vi "GetHWinfobyWMIC.vi"() -> (1 "CPUID":string, 2 "BoardSN":string)   [LabVIEW 2015]
uses:
  <vilib>/regexp/Match Regular Expression.xnode
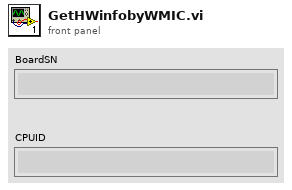
[diagram p1: front panel]
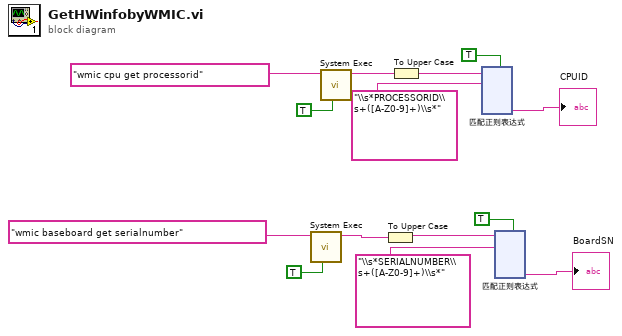
[diagram p0: block diagram]
diagram:
  n1 = call <vilib>:"System Exec.vi"("run minimized? (F)"=TRUE, "command line"="wmic baseboard get serialnumber") -> ("standard output"=w5:string)  [unwired: 6 in, 3 out]
  n2 = call <vilib>:"System Exec.vi"("run minimized? (F)"=TRUE, "command line"="wmic cpu get processorid") -> ("standard output"=w11:string)  [unwired: 6 in, 3 out]
  n3 = To Upper Case(1:w5) -> (0:w1:string)
  n4 = To Upper Case(1:w11) -> (0:w10:string)
  n5 = xnode "匹配正则表达式"("输入字符串"=w10, "正则表达式"="\\s*PROCESSORID\\s+([A-Z0-9]+)\\s*", "多行？(F)"=TRUE) -> ("子匹配 1"=→"CPUID":string)  [unwired: 3 in, 5 out]
  n6 = xnode "匹配正则表达式"("输入字符串"=w1, "正则表达式"="\\s*SERIALNUMBER\\s+([A-Z0-9]+)\\s*", "多行？(F)"=TRUE) -> ("子匹配 1"=→"BoardSN":string)  [unwired: 3 in, 5 out]
